vi "Read SP.vi"(8 "error in":errorcluster, 11 "Generic Init CVT Message in":refnum<class "Generic Init CVT Message.lvclass">) -> (0 "error out":errorcluster, 2 "SP":dbl, 3 "Generic Init CVT Message out":refnum<class "Generic Init CVT Message.lvclass">)   [LabVIEW 2014, in "DAQ Device.lvlib" / "Generic Init CVT Message.lvclass"]
uses:
  Generic Init CVT Message.lvclass
  Generic Init CVT Message.lvclass/Generic Init CVT Message.ctl
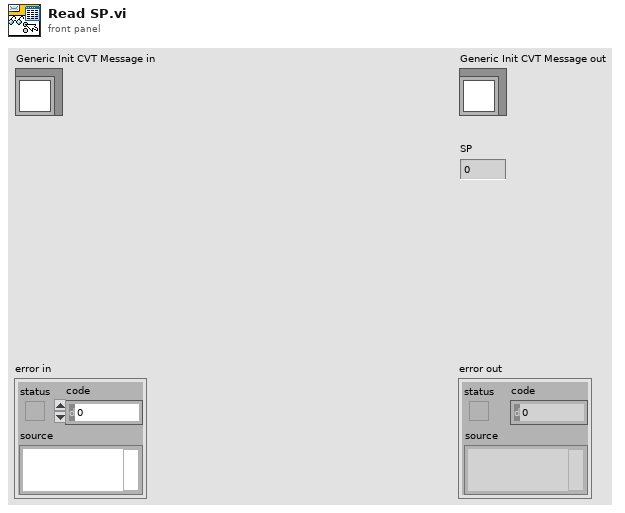
[diagram p1: front panel]
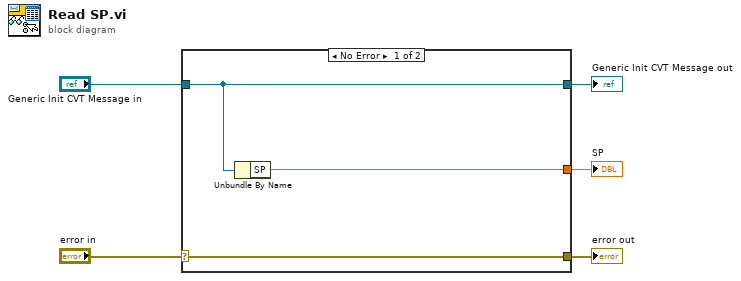
[diagram p0: block diagram]
diagram:
  n1 = case shown="No Error" "error in" {
    selector: "error in" -> [w8 w9]
    tunnel: [w8 w9] -> w4
    tunnel: [w7 w10] -> w2
    tunnel: "Generic Init CVT Message in" -> [w7 w10]
    tunnel: [w6 _] -> w1
    frame No Error {
      n2 = Unbundle By Name(w7) -> ("SP"=w6:dbl)
    }
    frame Error {
    }
  }
  "error out" <- w4
  "Generic Init CVT Message out" <- w2
  "SP" <- w1
